vi "db_transactions_selectFrom.vi"(0 "UDL PATH IN":path, 1 "TABLE NAME":string, 2 "FIELDS (*)":string[](array[string]), 3 "CONDITION":cluster{"FIELD":string, "VALUE":string}, 4 "MODE":bool, 5 "ERROR IN":errorcluster) -> (14 "UDL PATH OUT":path, 16 "RESULT":string[][](array[string]), 19 "ERROR OUT":errorcluster)   [LabVIEW 2018, in "db_lib R3.lvlib"]
uses:
  db_lib R3.lvlib
  <vilib>/addons/database/Connection.llb/DB Tools Open Connec (Path).vi
  <vilib>/addons/database/Connection.llb/Conn Execute.vi
  <vilib>/addons/database/Recordset.llb/Rec Fetch Recordset Data (R).vi
  <vilib>/addons/database/Recordset.llb/Rec Destroy - Connection.vi
  <vilib>/addons/database/_DB Variant To Data/Database Variant To Data.xnode
  <vilib>/addons/database/NI_Database_API.lvlib
panel:
  # "SELECT [fields] FROM [table_name] WHERE [condition];"
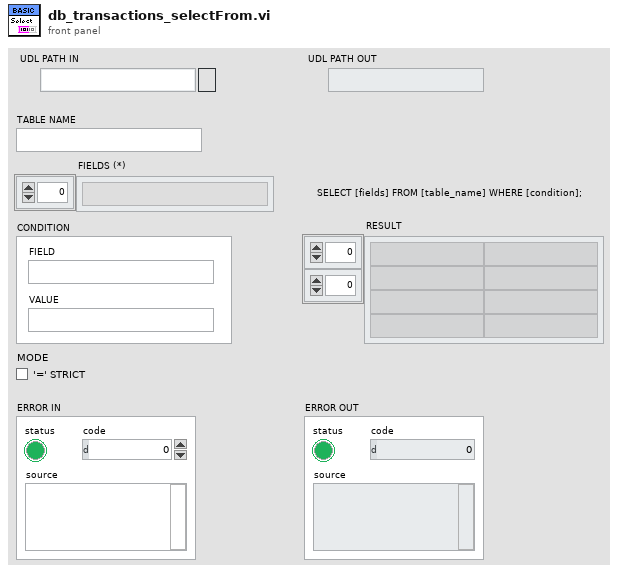
[diagram p1: front panel]
types:
  T1 = typedef "NI_Database_API.lvlib/Conn ObjectReference.ctl" = refnum<k1>
  T2 = typedef "NI_Database_API.lvlib/Rec ObjectReference.ctl" = refnum<k1>
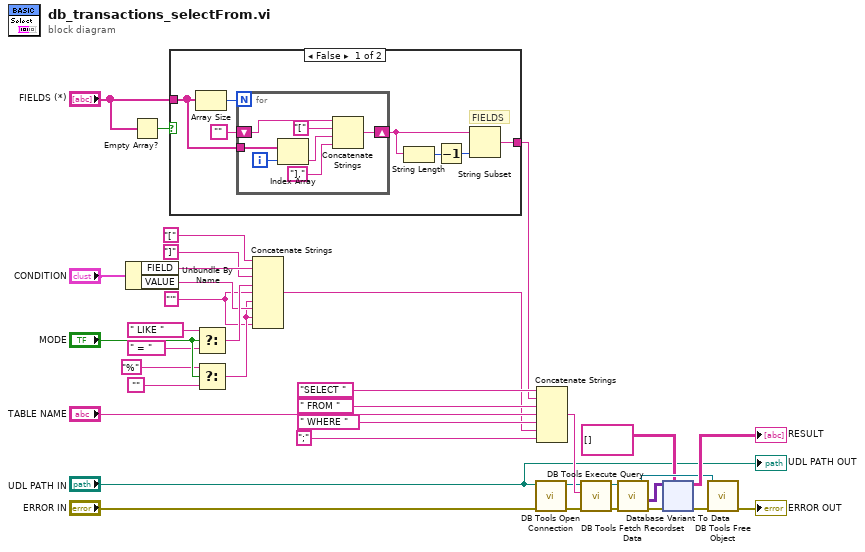
[diagram p0: block diagram]
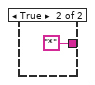
[diagram p2: hidden frame]
diagram:
  w10 = "'" ("string")
  n1 = Unbundle By Name("CONDITION") -> ("FIELD"=w19:string, "VALUE"=w12:string)
  n2 = Empty Array?(array="FIELDS (*)") -> (empty?=w22:bool)
  n3 = case shown="False" w22 {
    tunnel: "FIELDS (*)" -> [w38 _]
    tunnel: [w37 "*"] -> w21
    frame False {
      # "FIELDS"
      n4 = Array Size(array=w38) -> (size(s)=w39:i32)
      n5 = for {
        N: w39 -> [_]
        tunnel: w38 -> [w50]
        shift-right: [w45] -> w42
        shift-left: "" -> [w44]
        i -> [w49]
        n6 = Index Array(array=w50, index=w49) -> (element=w47:string)
        n7 = Concatenate Strings(w44, "[" ("string"), w47, "]," ("string")) -> (w45:string)
      }
      n8 = String Length(string=w42) -> (length=w41:i32)
      n9 = Decrement(x=w41) -> (x-1=w40:i32)
      n10 = String Subset(string=w42, length (rest)=w40) -> (substring=w37:string)  [unwired: 1 in]
    }
    frame True {
    }
  }
  n11 = Select(t=" LIKE ", s="MODE", f=" = ") -> (s? t:f=w16:string)
  n12 = Select(t="%", s="MODE", f="") -> (s? t:f=w11:string)
  n13 = Concatenate Strings("[" ("string"), w19, "]" ("string"), w16, w10, w11, w12, w11, w10) -> (w9:string)
  n14 = call-poly <vilib>:"DB Tools Open Connection.vi"("error in (no error)"="ERROR IN", "connection information"="UDL PATH IN") -> ("error out"=w7:errorcluster, "connection reference"=w6:T1)  [unwired: 6 in]
  n15 = Concatenate Strings("SELECT ", w21, " FROM ", "TABLE NAME", " WHERE ", w9, ";" ("string")) -> (w32:string)
  n16 = call-poly <vilib>:"DB Tools Execute Query.vi"("error in (no error)"=w7, "SQL query"=w32, "connection reference"=w6) -> ("error out"=w31:errorcluster, "recordset reference"=w30:T2)  [unwired: 5 in]
  n17 = call-poly <vilib>:"DB Tools Fetch Recordset Data.vi"("error in (no error)"=w31, "recordset reference"=w30) -> ("error out"=w28:errorcluster, "recordset data"=w27:variant[][], "recordset reference out"=w26:T2)  [unwired: 3 in]
  n18 = xnode "Database Variant To Data"("database variant"=w27, "error in (no error)"=w28, "type"=string[][] []) -> ("data"=→"RESULT":string[][], "error out"=w29:errorcluster)
  n19 = call-poly <vilib>:"DB Tools Free Object.vi"("error in (no error)"=w29, "recordset reference"=w26) -> ("error out"=→"ERROR OUT":errorcluster)  [unwired: 8 in, 1 out]
  "UDL PATH OUT" <- "UDL PATH IN"
